vi "OM3_CleaningGlobal.vi"() -> ()   [LabVIEW 2014]
panel:
  in  "odor#":i32
  out "cleaning done":bool
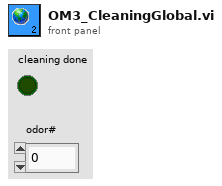
[diagram p1: front panel]
diagram:
